vi "FL Create Membership Function (User-Defined).vi"(0 "left base":dbl, 1 "name":string, 5 "left top":dbl, 7 "right top":dbl, 9 "right base":dbl, 11 "error in (no error)":errorcluster, 12 "color":u32(colorbox), 13 "user-defined membership function shapes":cluster{"Y":dbl[], "X":dbl[]}[](array[cluster]), 14 "user-defined shape index":i32) -> (4 "membership function":T1 {"shape" items=["Triangle", "Trapezoid", "Singleton", "Sigmoid", "Gaussian", "User-Defined"]}, 15 "error out":errorcluster)   [LabVIEW 2020, in "NI_Fuzzy_Logic_API.lvlib"]
doc: "Creates a membership function for a linguistic variable. You also can use the Define Variable dialog box to create membership functions interactively."
uses:
  <vilib>/addons/Fuzzy Logic/NI_Fuzzy_Logic_API.lvlib
  <vilib>/addons/Fuzzy Logic/TypeDefs/FL Membership Function.ctl
  <vilib>/addons/Fuzzy Logic/TypeDefs/FL Membership Function Shape.ctl
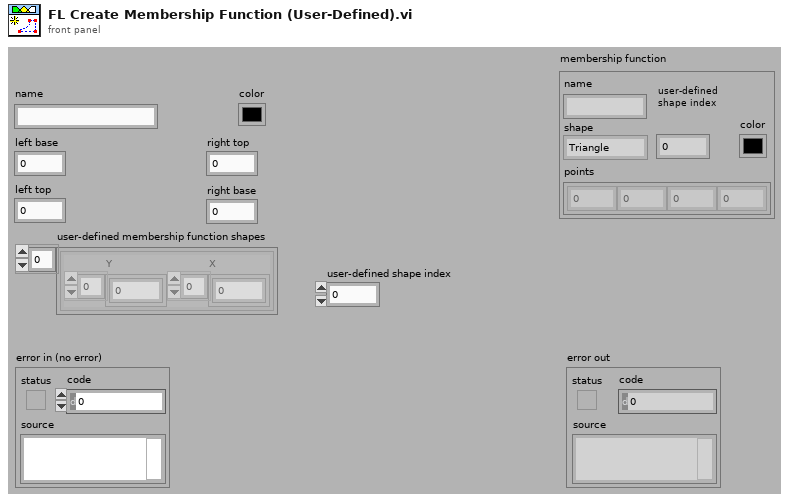
[diagram p1: front panel]
types:
  T1 = typedef "NI_Fuzzy_Logic_API.lvlib/FL Membership Function.ctl" = cluster{"name":string, "shape":T2, "points":dbl[], "color":u32, "user-defined shape index":i32}
  T2 = typedef "NI_Fuzzy_Logic_API.lvlib/FL Membership Function Shape.ctl" = u16
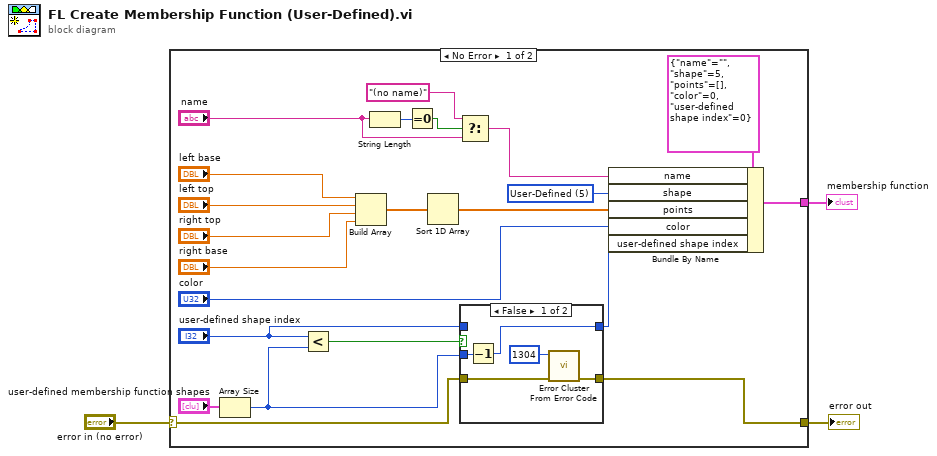
[diagram p0: block diagram]
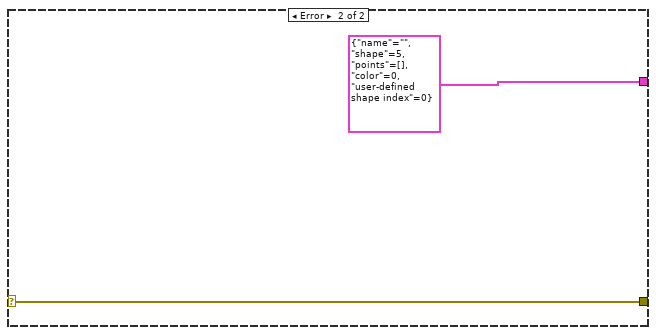
[diagram p3: hidden frame]
diagram:
  n1 = case shown="No Error" "error in (no error)" {
    selector: "error in (no error)" -> [w10 w34]
    tunnel: [w25 T1 {"name"="", "shape"=5, "points"=[], "color"=0, "user-defined shape index"=0} ("Membership Function")] -> w1
    tunnel: [w9 w34] -> w2
    frame No Error {
      w6 = T2 5 items=["Triangle", "Trapezoid", "Singleton", "Sigmoid", "Gaussian", "User-Defined"] ("shape")
      n2 = Array Size(array="user-defined membership function shapes") -> (size(s)=w8:i32)
      n3 = Less?(x="user-defined shape index", y=w8) -> (x < y?=w5:bool)
      n4 = Build Array("left base", "left top", "right top", "right base") -> (w18:dbl[])
      n5 = String Length(string="name") -> (length=w24:i32)
      n6 = Equal To 0?(x=w24) -> (x = 0?=w23:bool)
      n7 = Sort 1D Array(array=w18) -> (sorted array=w15:dbl[])
      n8 = Select(t="(no name)", s=w23, f="name") -> (s? t:f=w14:string)
      n9 = case shown="False" w5 {
        tunnel: "user-defined shape index" -> [_ w32]
        tunnel: [w26 w32] -> w4
        tunnel: w10 -> [w29 w31]
        tunnel: [w28 w31] -> w9
        tunnel: w8 -> [w27 _]
        frame False {
          n10 = Decrement(x=w27) -> (x-1=w26:i32)
          n11 = call <vilib>:"Error Cluster From Error Code.vi"("error in (no error)"=w29, "error code (0)"=1304) -> ("error out"=w28:errorcluster)  [unwired: 1 in, 6 out]
        }
        frame True {
        }
      }
      n12 = Bundle By Name(cluster=T1 {"name"="", "shape"=5, "points"=[], "color"=0, "user-defined shape index"=0} ("Membership Function"), "name"=w14, "shape"=w6, "points"=w15, "color"="color", "user-defined shape index"=w4) -> (w25:T1)
    }
    frame Error {
    }
  }
  "membership function" <- w1
  "error out" <- w2
